vi "Complete_Controller.vi"() -> ()   [LabVIEW 2014]
uses:
  <vilib>/Instr/_visa.llb/VISA Configure Serial Port (Instr).vi
  <vilib>/Utility/file.llb/Read From Spreadsheet File (string).vi
  <vilib>/DAQmx/read.llb/DAQmx Read (Analog 1D DBL NChan 1Samp).vi
  <vilib>/DAQmx/write.llb/DAQmx Write (Analog 1D DBL NChan 1Samp).vi
  <vilib>/DAQmx/write.llb/DAQmx Write (Digital Bool 1Line 1Point).vi
  Environmental Chamber LabVIEW and Instruments/Drivers and Software/keithley_6430/Keithley 6430/Public/Data/Read (Single Point).vi
  Environmental Chamber LabVIEW and Instruments/Drivers and Software/LabVIEW 8.2 Drivers/keithley_24xx/Keithley 24XX/Public/Data/Read (Single Point).vi
  <vilib>/Utility/file.llb/Write To Spreadsheet File (string).vi
  Environmental Chamber LabVIEW and Instruments/Drivers and Software/keithley_24xx/Keithley 24XX/Keithley 24XX.lvlib
  Environmental Chamber LabVIEW and Instruments/Drivers and Software/keithley_6430/Keithley 6430/Keithley 6430.lvlib
panel:
  in  "Turbo pump\nauto on":bool=TRUE
  in  "Use excel file\nfor sequence?":bool
  out "Sequence time left (hrs)":dbl caption="min"
  out "Sequence Preview":cluster{dbl[], dbl[]}[](graph)
  in  "Import sequence file":path
  out "Pressure Control 3":bool caption="Pressure Control"
  in  "valve % open":dbl=100.0 min=0.0 max=100.0 step=5.0
  out "Pressure Control 2":bool caption="Pressure Control"
  out "Keithley 6430":bool
  out "J-Kem":bool caption="J-Kem Temp"
  out "J-Kem Temp (C)":cluster{dbl}(graph)
  out "Keithley 2420":bool caption="Keithley 2430"
  out "Pressure Control":bool
  out "Arduino":bool
  out "temp\n(C)":string
  out "gas\nsensor":string
  out "Arduino humidity (%)":cluster{dbl}(graph)
  out "SRS QCM":bool
  out "MHz":dbl format="%.7f"
  out "Ohm":dbl format="%.4e"
  out "Waveform Chart 7":cluster{dbl, "Resistance out":dbl}(graph)
  out "Chamber Pressure (Torr)":cluster{"f":dbl}(graph)
  in  "Start recording after":dbl caption="min"
  in  "Auto stop after":bool
  in  "hrs":dbl=1000.0 min=0.0
  out "Start Time":string
  out "Elapsed (min)":dbl caption="Elapsed Time (s)"
  in  "Delay between data points (s)":dbl caption="sec" min=0.0 max=30.0 format="%#_13g"
  in  "Vapor\nflow\n(sccm)":sgl(slide) min=0 max=100 step=1 scale=0.0..100.0
  out "Actual":dbl
  out "Boolean 3":bool
  out "Actual":dbl
  out "Boolean":bool
  in  "Gas\nflow\n(sccm)":sgl(slide) min=0 max=100 step=1 scale=0.0..100.0
  in  "Turbo pump auto on":bool
  in  "Desired pressure":dbl min=0.0 max=760.0 step=5.0
  out "Valve position (%)":dbl
  in  "Pressure Control":enum32{"Open Mode (%)", "Pressure Mode (Torr)"}(radio)
  in  "stop":bool
  in  "Experiment Notes":string
  in  "Clear all charts":bool
  out "Save data file path":path
  out "Waveform Chart 2":cluster{"f":dbl, "f":dbl}(graph)
  out "Keithley 2420 (Ohm)":cluster{"Resistance":sgl}(graph)
  out "Keithley 6430 (Ohm)":cluster{"Measurement":dbl}(graph)
  in  "Tab Control":enum32{"Run Sequence", "Create Sequence"}(tab)
  out "User-defined\nsequence 2":string[][](table) caption="Sequence to run"
  in  "Run Sequence":bool
  out "Current step":i32
  out "Step time remaining (min)":dbl caption="min"
  in  "User-defined\nsequence":string[][](table) caption="Create sequence"
  out "QCM mass deposited (ug)":cluster{dbl}(graph)
  in  "rapidox O2 Sensor":bool
  in  "setnag O2 Pump":bool
  in  "Baud Rate 2":i32(ring)=2 items=["2400", "4800", "9600", "19200", "38400", "57600", "115200"]
  in  "Com Port":i32(ring) items=["Com 1", "Com 2", "Com 3", "Com 4", "Com 5", "Com 6", "COM 7", "COM 8", "COM 9", "COM 10", "COM 11", "COM 12", "com 13", "COM 14"]
  in  "Com Port 2":i32(ring) items=["Com 1", "Com 2", "Com 3", "Com 4", "Com 5", "Com 6", "COM 7", "COM 8", "COM 9", "COM 10", "COM 11", "COM 12", "com 13", "COM 14"]
  out "Torr":dbl
  out "%":dbl
  out "atm":dbl
  out "Waveform Chart":cluster{dbl}(graph)
  out "O2 Concentration (PPM)":dbl
  out "Waveform Chart 6":cluster{dbl}(graph)
  # "Currently Unused"
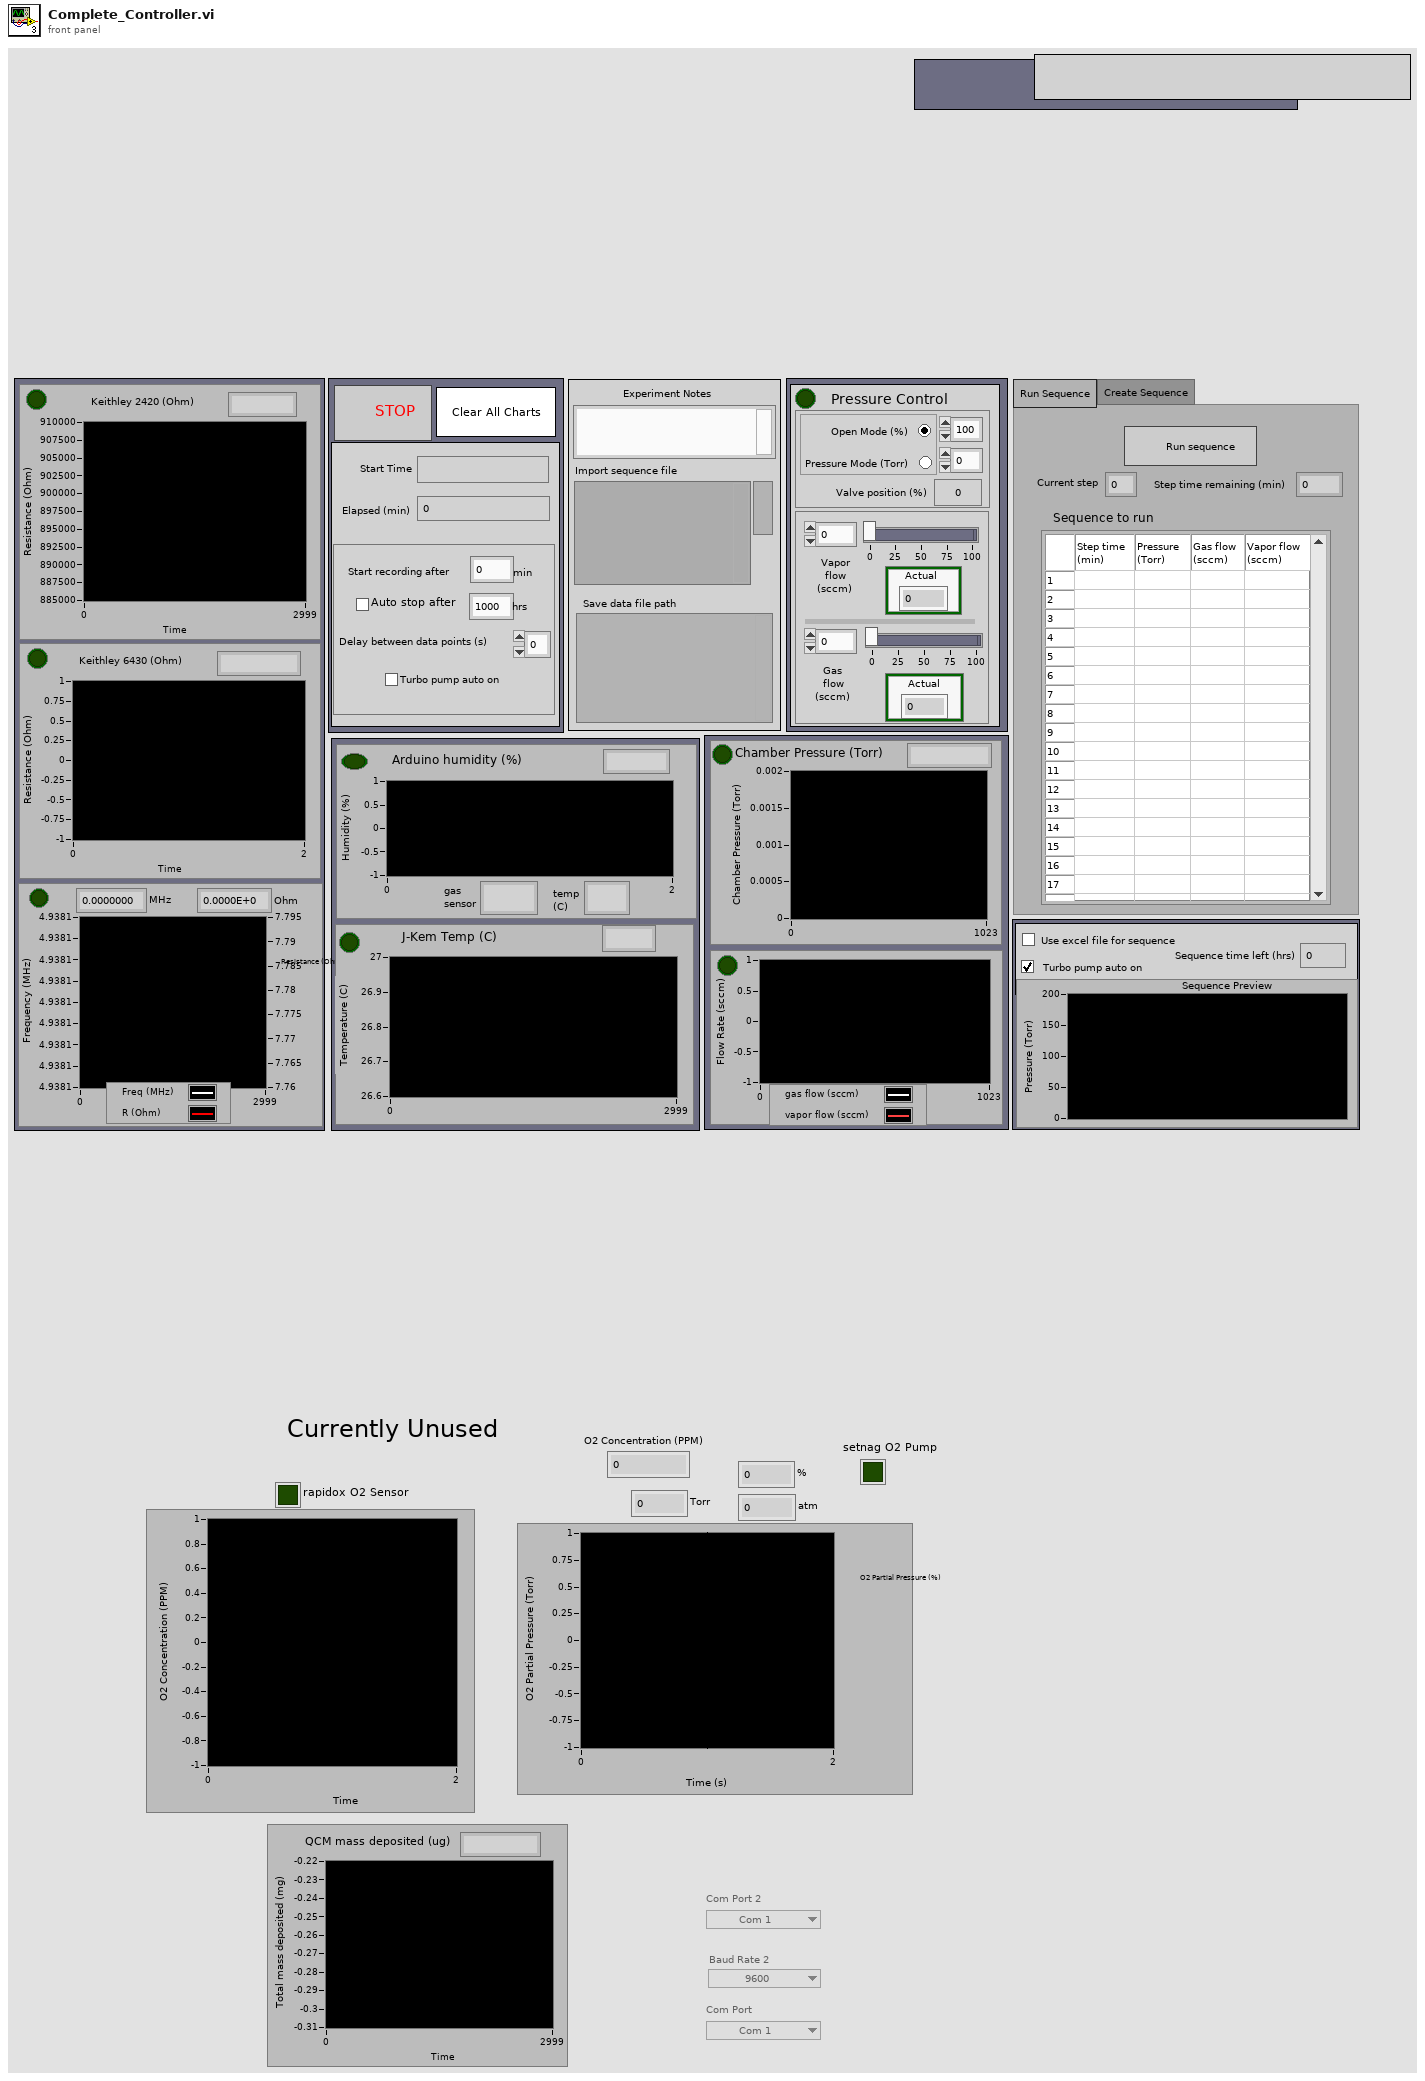
[diagram p1: front panel]
types:
  T1 = enum16{"open", "open or create", "create or replace", "create", "open (read only)"}
  T2 = enum16{"no parity", "odd parity", "even parity", "mark parity", "space parity"}
  T3 = cluster{bool, "VISA resource name":refnum<visa-resource-name>, "error out":errorcluster}
  T4 = cluster{bool, "VISA resource name out":refnum<visa-resource-name>, "error out":errorcluster}
  T5 = cluster{"task out":refnum<k21>, "error out":errorcluster, "task out":refnum<k21>, "error out":errorcluster, "task out":refnum<k21>, "error out":errorcluster, "VISA resource name":refnum<visa-resource-name>, "error out":errorcluster}
  T6 = cluster{"task out":refnum<k21>, "error out":errorcluster, "task out":refnum<k21>, "error out":errorcluster, "task out":refnum<k21>, "error out":errorcluster, "VISA resource name out":refnum<visa-resource-name>, "error out":errorcluster}
  T7 = cluster{bool, "VISA out":refnum<visa-resource-name>, "error out":errorcluster}
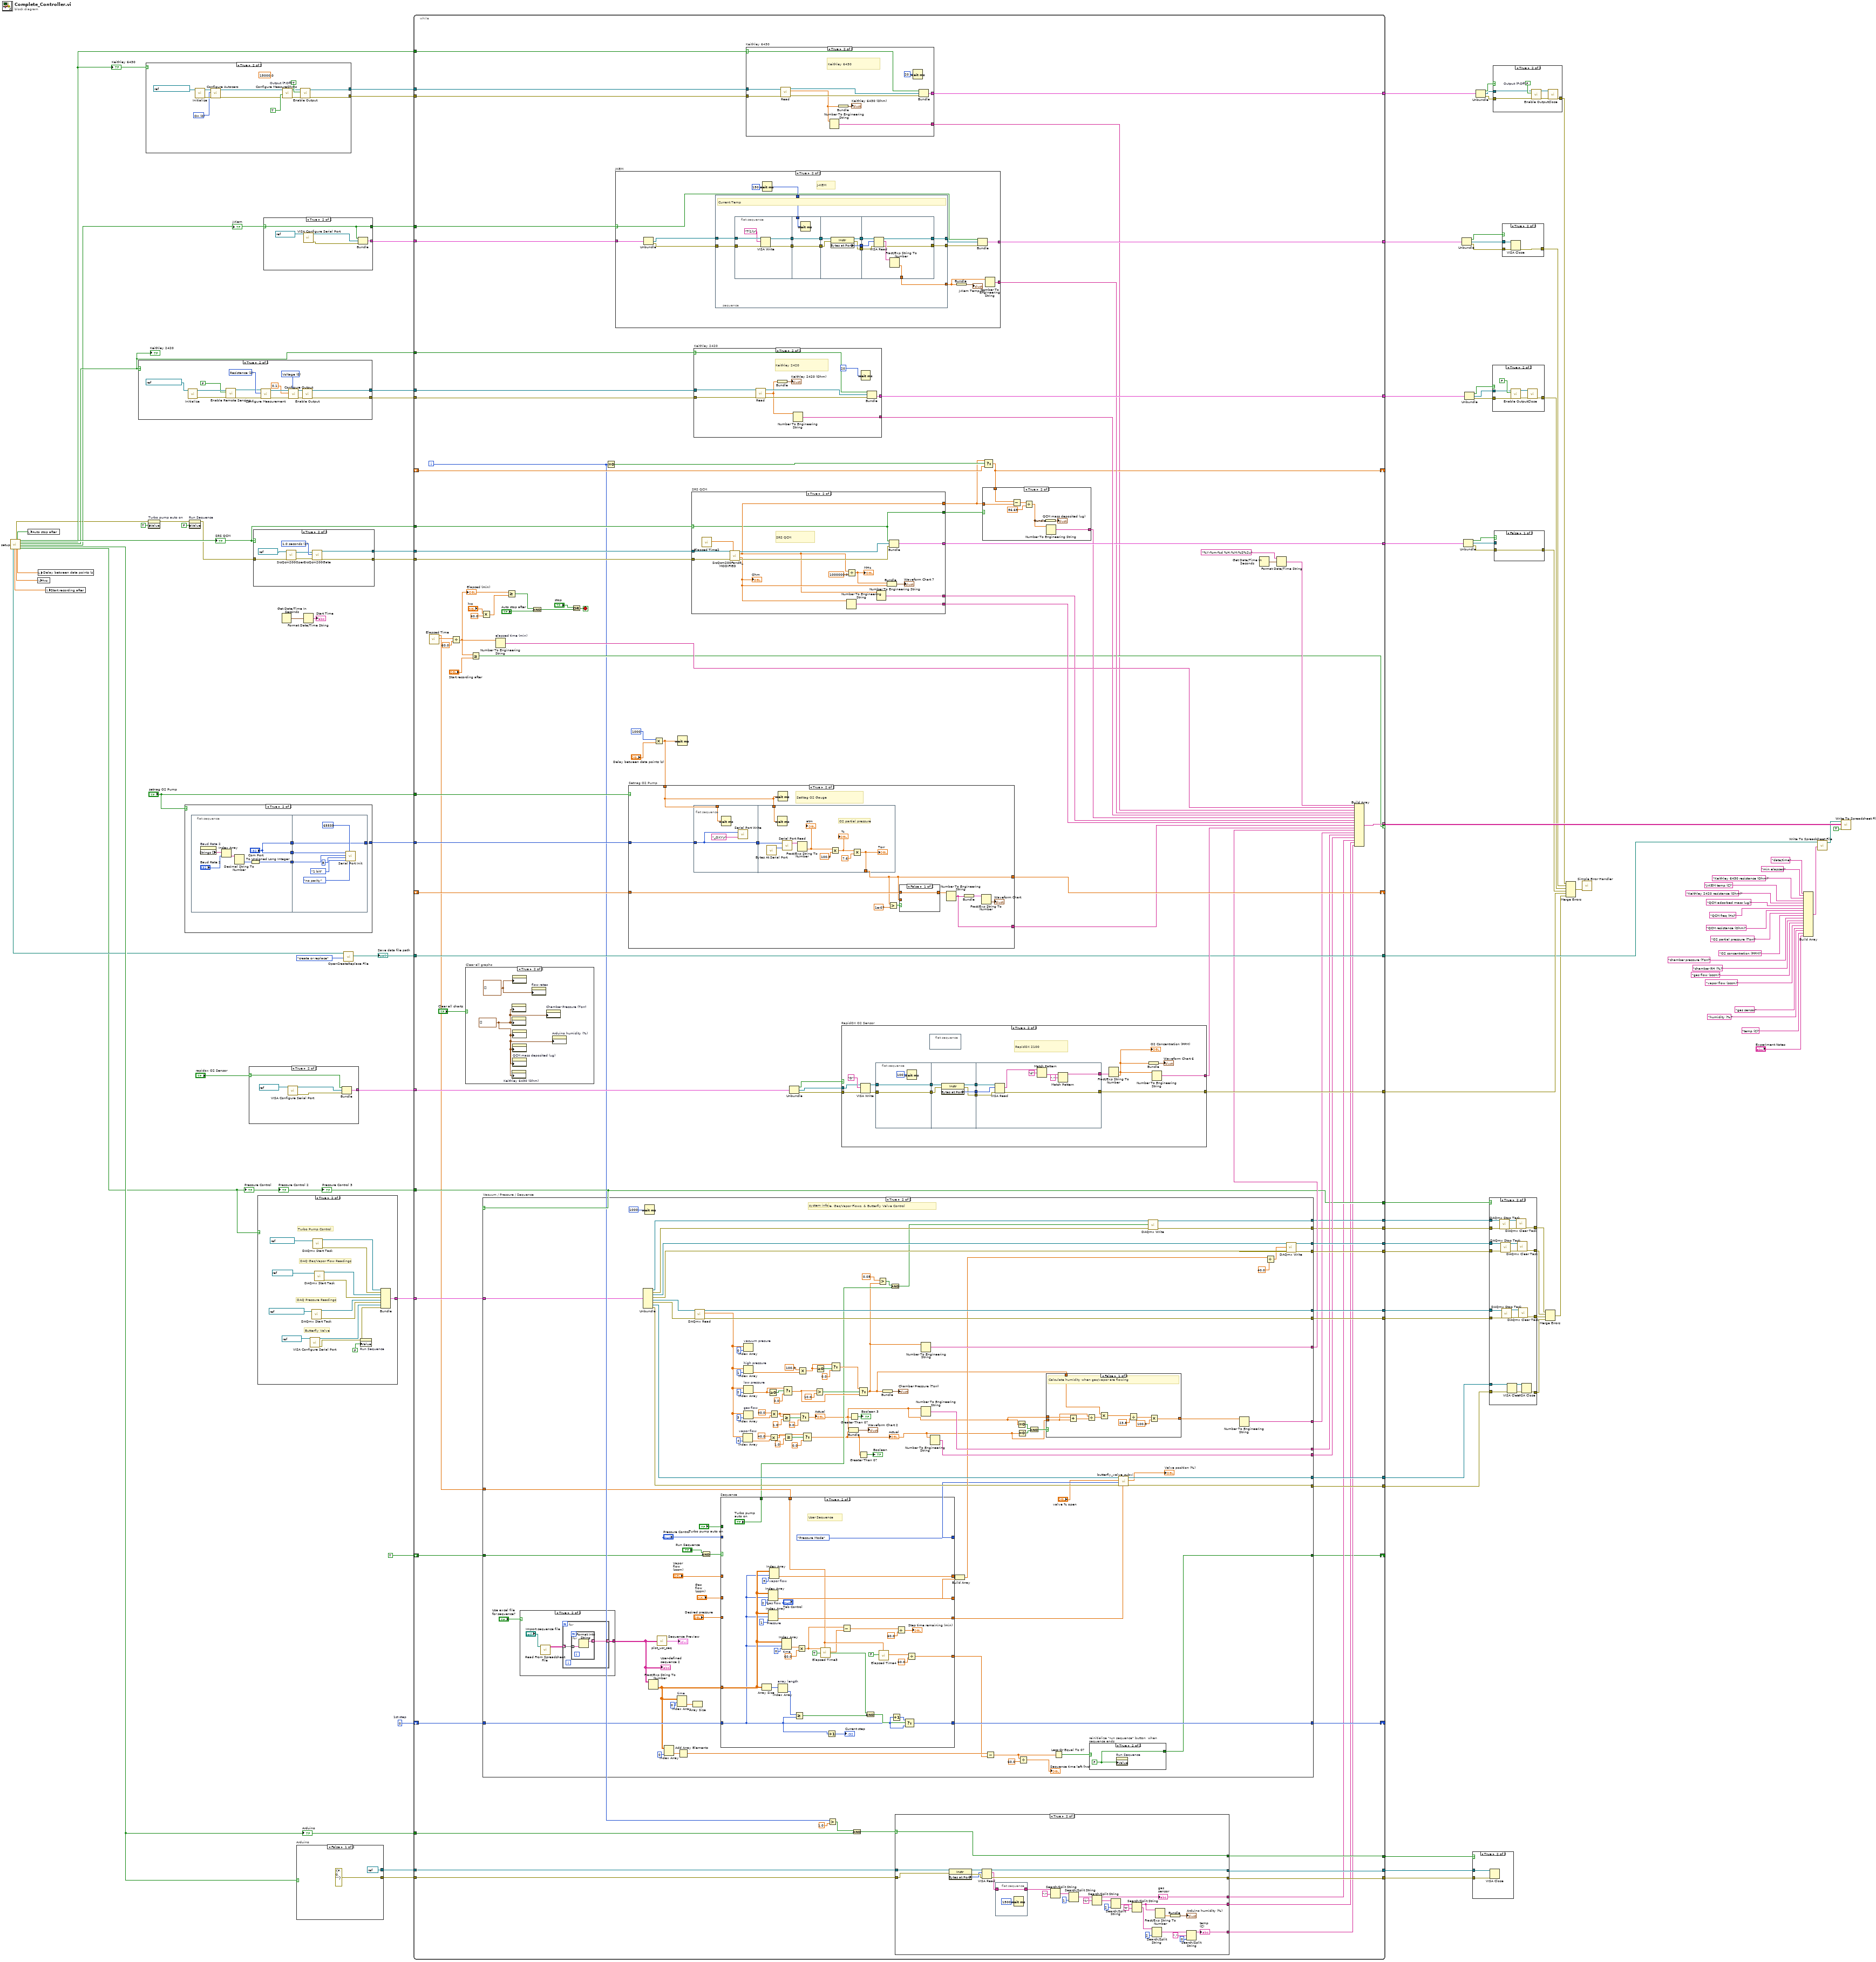
[diagram p0: block diagram]
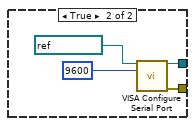
[diagram p3: hidden frame]
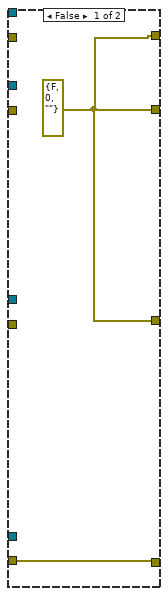
[diagram p4: hidden frame]
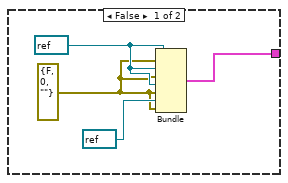
[diagram p5: hidden frame]
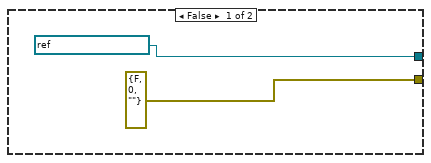
[diagram p7: hidden frame]
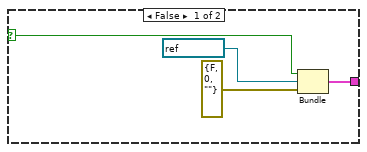
[diagram p8: hidden frame]
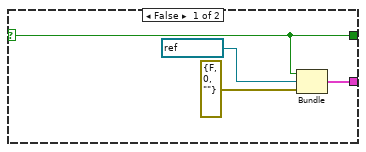
[diagram p10: hidden frame]
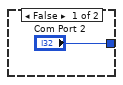
[diagram p11: hidden frame]
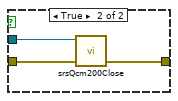
[diagram p12: hidden frame]
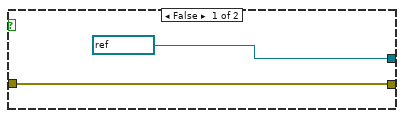
[diagram p13: hidden frame]
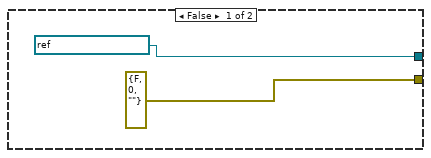
[diagram p15: hidden frame]
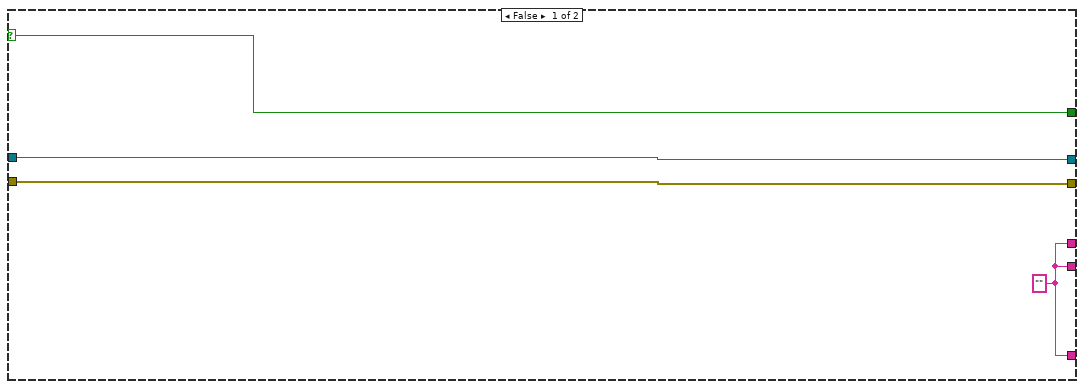
[diagram p16: hidden frame]
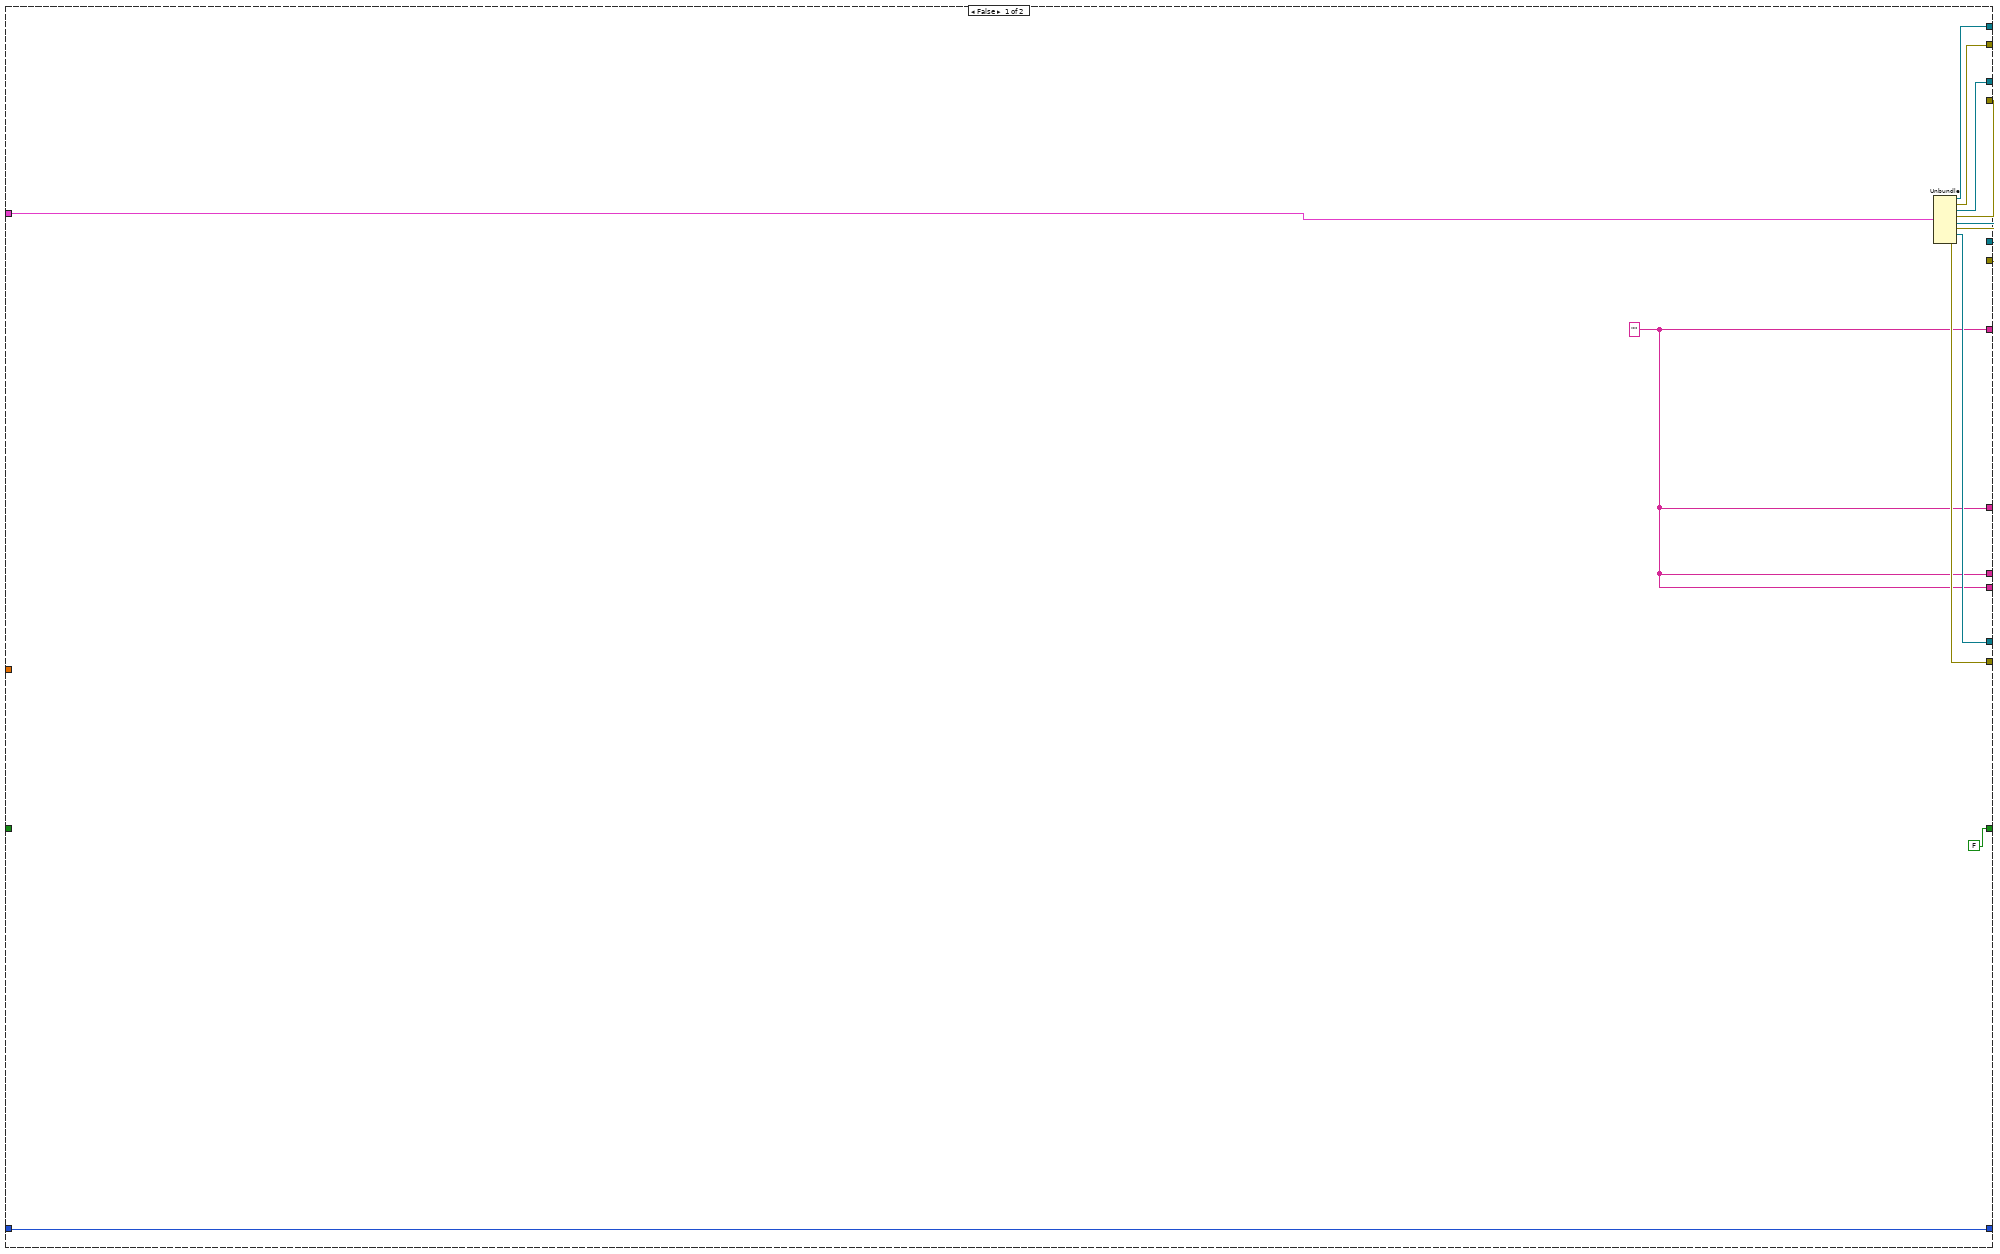
[diagram p17: hidden frame]
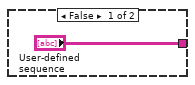
[diagram p18: hidden frame]
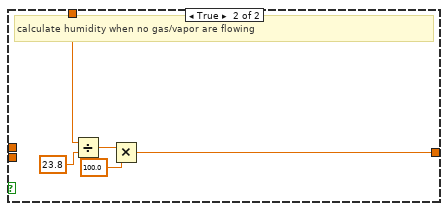
[diagram p19: hidden frame]
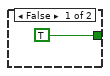
[diagram p20: hidden frame]
diagram:
  w29 = 0  # 1st step
  n1 = call "setup.vi"() -> ("Save file path 2"=w10:path, "begin recording"=w16:dbl, "error IO"=w3:errorcluster, "stop after"=w18:dbl, "Auto Stop 2"=w19:bool, "delay 5"=w17:dbl, "SRS QCM 2"=w15:bool, "Keithley 6431"=w11:bool, "Keithley 2421"=w14:bool, "J-KEM2"=w13:bool, "Arduino2"=w12:bool, "Pressure control 2"=w9:bool)  [unwired: 8 in]
  "SRS QCM" <- w15
  "Arduino" <- w12
  "Pressure Control" <- w9
  "Keithley 2420" <- w14
  "J-Kem" <- w13
  "Keithley 6430" <- w11
  "Pressure Control 2" <- w9
  "Pressure Control 3" <- w9
  n2 = local write "Auto stop after"(w19) -> ()
  n3 = local write "hrs"(w18) -> ()
  n4 = local write "Delay between data points (s)"(w17) -> ()
  n5 = local write "Start recording after"(w16) -> ()
  n6 = case shown="True" w14 {
    tunnel: [refnum<visa-resource-name> "GPIB1::24::INSTR" ("VISA resource name") w108] -> w96
    tunnel: [errorcluster {"status"=FALSE, "code"=0, "source"=""} ("error out") w103] -> w95
    frame False {
    }
    frame True {
      w110 = u16 0 items=["Voltage", "Current"] ("Source Mode  (0: Voltage)")
      w115 = u16 2 items=["Volts", "Current", "Resistance"] ("Function (0: Volts)")
      n7 = call "Initialize.vi"("VISA resource name"=refnum<visa-resource-name> "GPIB1::24::INSTR") -> ("error out"=w104:errorcluster, "VISA resource name out"=w107:refnum<visa-resource-name>)  [unwired: 9 in]
      n8 = call "Enable Remote Sensing.vi"("error in (no error)"=w104, "Enable Remote Sensing (T: Enable)"=FALSE ("4-wire?"), "VISA resource name"=w107) -> ("error out"=w105:errorcluster, "VISA resource name out"=w106:refnum<visa-resource-name>)  [unwired: 7 in]
      n9 = call "Configure Measurement.vi"("error in (no error)"=w105, "Function (0: Volts)"=w115, "VISA resource name"=w106) -> ("error out"=w114:errorcluster, "VISA resource name out"=w113:refnum<visa-resource-name>)  [unwired: 7 in]
      n10 = call "Configure Output.vi"("Source Mode  (0: Voltage)"=w110, "error in (no error)"=w114, "Output Level (0)"=0.1 ("Applied Voltage (V)"), "VISA resource name"=w113) -> ("error out"=w112:errorcluster, "VISA resource name out"=w111:refnum<visa-resource-name>)  [unwired: 6 in]
      n11 = call "Enable Output.vi"("error in (no error)"=w112, "VISA resource name"=w111) -> ("error out"=w103:errorcluster, "VISA resource name out"=w108:refnum<visa-resource-name>)  [unwired: 8 in]
    }
  }
  n12 = case shown="True" w11 {
    tunnel: [refnum<visa-resource-name> "GPIB0::29::INSTR" ("VISA resource name") w125] -> w53
    tunnel: [errorcluster {"status"=FALSE, "code"=0, "source"=""} ("error out") w126] -> w52
    frame False {
    }
    frame True {
      (unwired) 15000.0 ("Resistance Range [Ohms]")
      w121 = u16 0 items=["On", "Off", "Once"] ("Autozero  (0: On)")
      w129 = TRUE  # Output (F:Off)
      n13 = call "Initialize.vi"("VISA resource name"=refnum<visa-resource-name> "GPIB0::29::INSTR") -> ("error out"=w122:errorcluster, "VISA resource name out"=w123:refnum<visa-resource-name>)  [unwired: 4 in, 5 out]
      n14 = call "Configure Autozero.vi"("error in (no error)"=w122, "Autozero  (0: On)"=w121, "VISA resource name"=w123) -> ("error out"=w119:errorcluster, "VISA resource name out"=w120:refnum<visa-resource-name>)  [unwired: 7 in]
      n15 = call "Configure MeasureOhms.vi"("error in (no error)"=w119, "Auto Range (T:Enable)"=TRUE, "VISA resource name"=w120) -> ("error out"=w130:errorcluster, "VISA resource name out"=w128:refnum<visa-resource-name>)  [unwired: 3 in, 4 out]
      n16 = call "Enable Output.vi"("error in (no error)"=w130, "Enable Output (F:Off)"=w129, "VISA resource name"=w128) -> ("error out"=w126:errorcluster, "VISA resource name out"=w125:refnum<visa-resource-name>)  [unwired: 7 out]
    }
  }
  n17 = property on="Turbo pump auto on" class="Bool (strict)"(error in=w3, "Value"=TRUE ("Turbo\npump")) -> (error out=w2:errorcluster)  [unwired: 1 in, 1 out]
  n18 = case shown="True" "setnag O2 Pump" {
    tunnel: ["Com Port 2" w132] -> w92
    frame False {
    }
    frame True {
      n19 = flat-sequence {
        tunnel: ["Com Port"] -> w135
        tunnel: [w137] -> w134
        tunnel: ["Com Port"] -> w133
        tunnel: w135 -> [w143]
        tunnel: w134 -> [w142]
        tunnel: w133 -> [w144]
        tunnel: [w144] -> w132
        frame #0 {
          n20 = property on="Baud Rate 2" class="Ring (strict)"() -> ("Strings []"=w139:string[])  [unwired: 2 in, 2 out]
          n21 = Index Array(array=w139, index="Baud Rate 2") -> (element=w140:string)
          n22 = Decimal String To Number(string=w140) -> (number=w138:i32)  [unwired: 2 in, 1 out]
          n23 = To Unsigned Long Integer(number=w138) -> (unsigned 32bit integer=w137:u32)
        }
        frame #1 {
          n24 = call <vilib>:"Serial Port Init.vi"("parity"=T2."no parity", "buffer size"=u16 65535, "stop bits"=enum16{"1 bit", "1.5 bits", "2 bits"}."1 bit", "data bits"=u16 8, "baud rate"=w142, "port number"=w143) -> ()  [unwired: 1 in, 1 out]
        }
      }
    }
  }
  n25 = property on="Run Sequence" class="Bool (strict)"(error in=w2, "Value"=FALSE ("Run Sequence")) -> (error out=w7:errorcluster)  [unwired: 1 in, 1 out]
  n26 = case shown="True" "rapidox O2 Sensor" {
    selector: "rapidox O2 Sensor" -> [w149 w154]
    tunnel: [w150 w155] -> w63
    frame False {
      n27 = Bundle(w149, "VISA resource name"=refnum<visa-resource-name> "COM7", "error out"=errorcluster {"status"=FALSE, "code"=0, "source"=""}) -> (w150:T3)  [unwired: 1 in]
    }
    frame True {
      n28 = call-poly "VISA Configure Serial Port"("VISA resource name"=refnum<visa-resource-name> "COM7") -> ("VISA resource name out"=w156:refnum<visa-resource-name>, "error out"=w153:errorcluster)  [unwired: 13 in]
      n29 = Bundle(w154, "VISA resource name out"=w156, "error out"=w153) -> (w155:T4)  [unwired: 1 in]
    }
  }
  n30 = case shown="True" w15 {
    tunnel: [refnum<visa-resource-name> "COM6" ("VISA in") w162] -> w94
    tunnel: [w158 w161] -> w93
    tunnel: w7 -> [w158 w160]
    frame False {
    }
    frame True {
      w166 = u16 1 items=["0.1 seconds", "1.0 seconds", "10.0 seconds"] ("Gate in")
      n31 = call "SrsQcm200Open.vi"("error in"=w160, "VISA in"=refnum<visa-resource-name> "COM6") -> ("error out"=w163:errorcluster, "VISA out"=w164:refnum<visa-resource-name>)  [unwired: 3 in]
      n32 = call "SrsQcm200Gate.vi"("VISA in"=w164, "Gate in"=w166, "error in (no error)"=w163) -> ("VISA out"=w162:refnum<visa-resource-name>, "error out"=w161:errorcluster)  [unwired: 14 in, 1 out]
    }
  }
  n33 = case shown="True" w9 {
    tunnel: [w167 w174] -> w34
    frame False {
      w169 = refnum<k21> refnum ("task out")
      w168 = errorcluster {"status"=FALSE, "code"=0, "source"=""} ("error out")
      n34 = Bundle("task out"=w169, "error out"=w168, "task out"=w169, "error out"=w168, "task out"=w169, "error out"=w168, "VISA resource name"=refnum<visa-resource-name> refnum, "error out"=w168) -> (w167:T5)  [unwired: 1 in]
    }
    frame True {
      # "Turbo Pump Control"
      # "DAQ Gas/Vapor Flow Readings"
      # "DAQ Pressure Readings"
      # "Butterfly Valve"
      n35 = call-poly "VISA Configure Serial Port"("VISA resource name"=refnum<visa-resource-name> "COM5") -> ("VISA resource name out"=w175:refnum<visa-resource-name>, "error out"=w171:errorcluster)  [unwired: 13 in]
      n36 = call <vilib>:"DAQmx Start Task.vi"("task/channels in"=refnum<k21> "AllDaqReadings") -> ("task out"=w177:refnum<k21>, "error out"=w176:errorcluster)  [unwired: 13 in]
      n37 = call <vilib>:"DAQmx Start Task.vi"("task/channels in"=refnum<k21> "TurboON") -> ("task out"=w181:refnum<k21>, "error out"=w180:errorcluster)  [unwired: 13 in]
      n38 = call <vilib>:"DAQmx Start Task.vi"("task/channels in"=refnum<k21> "Setflow") -> ("task out"=w179:refnum<k21>, "error out"=w178:errorcluster)  [unwired: 13 in]
      n39 = property on="Run Sequence" class="Bool (strict)"(error in=w171, "Value"=FALSE ("Run Sequence")) -> (error out=w173:errorcluster)  [unwired: 1 in, 1 out]
      n40 = Bundle("task out"=w181, "error out"=w180, "task out"=w179, "error out"=w178, "task out"=w177, "error out"=w176, "VISA resource name out"=w175, "error out"=w173) -> (w174:T6)  [unwired: 1 in]
    }
  }
  n41 = case shown="True" w13 {
    selector: w13 -> [w186 w191]
    tunnel: [w187 w192] -> w81
    tunnel: [w186 w191] -> w75
    frame False {
      n42 = Bundle(w186, "VISA resource name"=refnum<visa-resource-name> "COM3", "error out"=errorcluster {"status"=FALSE, "code"=0, "source"=""}) -> (w187:T3)  [unwired: 1 in]
    }
    frame True {
      n43 = call-poly "VISA Configure Serial Port"("VISA resource name"=refnum<visa-resource-name> "COM3") -> ("VISA resource name out"=w193:refnum<visa-resource-name>, "error out"=w190:errorcluster)  [unwired: 13 in]
      n44 = Bundle(w191, "VISA resource name out"=w193, "error out"=w190) -> (w192:T4)  [unwired: 1 in]
    }
  }
  n45 = Get Date/Time In Seconds() -> (seconds since 1Jan1904=w99:timestamp)
  n46 = case "Arduino" shown="False" w12 {
    tunnel: [refnum<visa-resource-name> refnum ("VISA resource name out") w200] -> w28
    tunnel: [errorcluster {"status"=FALSE, "code"=0, "source"=""} ("error out") w197] -> w27
    frame False {
    }
    frame True {
      n47 = call-poly "VISA Configure Serial Port"("VISA resource name"=refnum<visa-resource-name> "COM12", "baud rate (9600)"=u32 9600) -> ("VISA resource name out"=w200:refnum<visa-resource-name>, "error out"=w197:errorcluster)  [unwired: 12 in]
    }
  }
  n48 = Format Date/Time String(seconds (now)=w99) -> (date/time string=→"Start Time":string)  [unwired: 2 in]
  n49 = call "OpenCreateReplace File.vi"("function (open:0)"=T1."create or replace", "file path"=w10) -> ("new file path"=w20:path)  [unwired: 6 in, 3 out]
  "Save data file path" <- w20
  n50 = while {
    shift-right: [w290] -> _
    shift-left: _ -> [w289]
    tunnel: [w219] -> w97 mode=indexing if=w218
    tunnel: w14 -> [w258]
    tunnel: w96 -> [w287]
    tunnel: w95 -> [w286]
    tunnel: w94 -> [w285]
    tunnel: w93 -> [w284]
    tunnel: w15 -> [w282]
    tunnel: "setnag O2 Pump" -> [w275]
    tunnel: w92 -> [w281]
    tunnel: [w277] -> w89
    tunnel: [w276] -> w85
    tunnel: w81 -> [w274]
    tunnel: [w273] -> w80
    tunnel: w75 -> [w271]
    tunnel: w63 -> [w267]
    tunnel: [w262] -> w61
    tunnel: [w257] -> w60
    tunnel: w20 -> [w257]
    shift-right: [w240] -> _
    shift-left: _ -> [w242]
    tunnel: w53 -> [w254]
    tunnel: w52 -> [w253]
    tunnel: [w252] -> w51
    tunnel: w11 -> [w251]
    tunnel: w9 -> [w232]
    tunnel: [w248] -> w47
    tunnel: [w247] -> w44
    tunnel: [w246] -> w46
    tunnel: [w245] -> w45
    tunnel: [w232] -> w43
    tunnel: [w244] -> w38
    tunnel: w34 -> [w236]
    tunnel: [w235] -> w32
    tunnel: [w234] -> w31
    tunnel: [w233] -> w30
    shift-right: [w231] -> _
    shift-left: w29 -> [w230]
    tunnel: w12 -> [w215]
    tunnel: w28 -> [w225]
    tunnel: w27 -> [w224]
    tunnel: [w223] -> w26
    tunnel: [w222] -> w25
    tunnel: [w221] -> w24
    shift-right: [w206] -> _
    shift-left: TRUE -> [w207]
    i -> [w204]
    stop <- w270 stop-if-true
    n51 = call "Elapsed Time"() -> ("Present (s)"=w229:dbl, "Elapsed Time (s)"=w269:dbl)  [unwired: 12 in, 6 out]
    n52 = Divide(x=w269, y=60.0) -> (x/y=w209:dbl)
    "Elapsed (min)" <- w209
    n53 = case "Clear all graphs" shown="True" "Clear all charts" {
      frame False {
      }
      frame True {
        w529 = cluster{dbl, "Resistance out":dbl}[] [] ("History Data")
        w528 = cluster{dbl}[] [] ("History Data")
        n54 = property on="Keithley 2420 (Ohm)" class="WFChart (strict)"("History Data"=w528) -> ()  [unwired: 2 in, 2 out]
        n55 = property on="J-Kem Temp (C)" class="WFChart (strict)"("History Data"=w528) -> ()  [unwired: 2 in, 2 out]
        n56 = property on="Keithley 6430 (Ohm)" class="WFChart (strict)"("History Data"=w528) -> ()  [unwired: 2 in, 2 out]
        n57 = property on="Waveform Chart 7" class="WFChart (strict)"("History Data"=w529) -> ()  [unwired: 2 in, 2 out]
        n58 = property on="Waveform Chart" class="WFChart (strict)"("History Data"=w528) -> ()  [unwired: 2 in, 2 out]
        n59 = property on="Waveform Chart 6" class="WFChart (strict)"("History Data"=w528) -> ()  [unwired: 2 in, 2 out]
        n60 = property on="QCM mass deposited (ug)" class="WFChart (strict)"("History Data"=w528) -> ()  [unwired: 2 in, 2 out]
        n61 = property on="flow rates" class="WFChart (strict)"("History Data"=w529) -> ()  [unwired: 2 in, 2 out]
        n62 = property on="Chamber Pressure (Torr)" class="WFChart (strict)"("History Data"=w528) -> ()  [unwired: 2 in, 2 out]
        n63 = property on="Arduino humidity (%)" class="WFChart (strict)"("History Data"=w528) -> ()  [unwired: 2 in, 2 out]
      }
    }
    n64 = Greater Or Equal?(x=w209, y="Start recording after") -> (x >= y?=w218:bool)
    n65 = Multiply(x="hrs", y=60.0) -> (x*y=w201:dbl)
    n66 = case "Vacuum / Pressure / Sequence" shown="True" w232 {
      tunnel: [w332 w439] -> w247
      tunnel: [w333 w438] -> w245
      tunnel: [w335 w419] -> w248
      tunnel: [w334 w420] -> w246
      tunnel: [w333 w410] -> w244
      tunnel: [w328 w400] -> w239
      tunnel: [w328 w399] -> w238
      tunnel: [w328 w397] -> w237
      tunnel: w236 -> [w338 w395]
      tunnel: [w337 w386] -> w235
      tunnel: [w336 w385] -> w234
      tunnel: [w331 w384] -> w233
      tunnel: w230 -> [w330 w366]
      tunnel: [w330 w381] -> w231
      tunnel: w229 -> [_ w380]
      tunnel: w207 -> [_ w357]
      tunnel: [FALSE ("new element/subarray") w352] -> w206
      tunnel: [w328 w351] -> w205
      frame False {
        w328 = ""
        n67 = Unbundle(w338) -> ("task out"=w337:refnum<k21>, "error out"=w336:errorcluster, "task out"=w335:refnum<k21>, "error out"=w334:errorcluster, "task out"=w332:refnum<k21>, "error out"=w333:errorcluster, "VISA resource name out"=w331:refnum<visa-resource-name>)  [unwired: 1 out]
      }
      frame True {
        # "system info"
        # "DAQ Pressure, Gas/Vapor Flows, & Butterfly Valve Control"
        n68 = case shown="True" "Use excel file\nfor sequence?" {
          tunnel: ["User-defined\nsequence" w442] -> w343
          frame False {
          }
          frame True {
            n69 = call-poly <vilib>:"Read From Spreadsheet File.vi"("file path (dialog if empty)"="Import sequence file") -> ("all rows"=w444:string[][])  [unwired: 6 in, 4 out]
            n70 = for {
              tunnel: w444 -> [w446] mode=indexing
              tunnel: [w445] -> w442 mode=indexing
              n71 = for {
                tunnel: w446 -> [w448] mode=indexing
                tunnel: [w447] -> w445 mode=indexing
                n72 = Format Into String(w448) -> (resulting string=w447:string)  [unwired: 3 in, 1 out]
              }
            }
          }
        }
        "User-defined\nsequence 2" <- w343
        n73 = Unbundle(w395) -> ("task out"=w388:refnum<k21>, "error out"=w387:errorcluster, "task out"=w389:refnum<k21>, "error out"=w390:errorcluster, "task out"=w391:refnum<k21>, "error out"=w392:errorcluster, "VISA resource name out"=w393:refnum<visa-resource-name>, "error out"=w394:errorcluster)
        n74 = Wait (ms)(milliseconds to wait=u32 1000) -> ()  [unwired: 1 out]
        n75 = Fract/Exp String To Number(string=w343) -> (number=w356:dbl[][])  [unwired: 3 in, 1 out]
        n76 = call "plot_usr_seq.vi"("User-defined sequence"=w343) -> ("Sequence Preview"=→"Sequence Preview":cluster{dbl[], dbl[]}[])
        n77 = Index Array(array=w356, index (col)=0 ("disabled index (col)")) -> (element=w370:dbl[])  [unwired: 1 in]
        n78 = Index Array "time"(array=w356, index (row)=0 ("disabled index (col)")) -> (element=w355:dbl[])  [unwired: 1 in]
        n79 = Add Array Elements(numeric array=w370) -> (sum=w361:dbl)
        n80 = Array Size(array=w355) -> ()  [unwired: 1 out]
        n81 = call-poly <vilib>:"DAQmx Read.vi"("task/channels in"=w391, "error in"=w392) -> ("task out"=w439:refnum<k21>, "data"=w430:dbl[], "error out"=w438:errorcluster)  [unwired: 11 in]
        n82 = And(x="Run Sequence", y=w357) -> (x .and. y?=w358:bool)
        n83 = case "Sequence" shown="True" w358 {
          tunnel: w380 -> [_ w487]
          tunnel: [w472 w488] -> w381
          tunnel: w366 -> [w472 w474]
          tunnel: "Vapor\nflow\n(sccm)" -> [w471 _]
          tunnel: "Gas\nflow\n(sccm)" -> [w470 _]
          tunnel: [w471 w496] -> w377
          tunnel: [w470 w495] -> w376
          tunnel: [w468 w494] -> w362
          tunnel: "Desired pressure" -> [w468 _]
          tunnel: "Turbo pump auto on" -> [w469 _]
          tunnel: [w469 "Turbo pump\nauto on"] -> w372
          tunnel: w356 -> [_ w481]
          tunnel: "Pressure Control" -> [w467 _]
          tunnel: [w467 enum32{"Open Mode", "Pressure Mode"}."Pressure Mode" ("Pressure Control")] -> w367
          tunnel: [0.0 w484] -> w360
          frame False {
          }
          frame True {
            # "User Sequence"
            n84 = Array Size(array=w481) -> (size(s)=w504:i32[])
            n85 = Index Array "gas flow"(array=w481, index (row)=w474, index (col)=2 ("disabled index (col)")) -> (element=w495:dbl)
            n86 = Index Array "Pressure"(array=w481, index (row)=w474, index (col)=1 ("disabled index (col)")) -> (element=w494:dbl)
            n87 = Index Array "vapor flow"(array=w481, index (row)=w474, index (col)=3 ("disabled index (col)")) -> (element=w496:dbl)
            n88 = Index Array "array length"(array=w504) -> (element=w482:i32)  [unwired: 1 in]
            n89 = Index Array "time"(array=w481, index (row)=w474, index (col)=0) -> (element=w493:dbl)
            n90 = Greater Or Equal?(x=w482, y=w474) -> (x >= y?=w501:bool)
            n91 = Multiply(x=w493, y=60.0) -> (x*y=w479:dbl)
            n92 = call "Elapsed Time3"("Time Target (s)"=w479, "Auto Reset"=TRUE, "Set Start Time (s)"=w487) -> ("Elapsed Time (s)"=w478:dbl, "Time has Elapsed"=w500:bool)  [unwired: 9 in, 6 out]
            n93 = Increment(x=w474) -> (x+1=→"Current step":i32)
            n94 = Subtract(x=w479, y=w478) -> (x-y=w475:dbl)
            n95 = And(x=w500, y=w501) -> (x .and. y?=w490:bool)
            n96 = call "Elapsed Time4"("Reset"=FALSE, "Set Start Time (s)"=w487) -> ("Elapsed Time (s)"=w485:dbl)  [unwired: 10 in, 7 out]
            n97 = Increment(x=w474) -> (x+1=w489:i32)
            n98 = Divide(x=w475, y=60.0) -> (x/y=→"Step time remaining (min)":dbl)
            n99 = Select(t=w489, s=w490, f=w474) -> (s? t:f=w488:i32)
            n100 = Divide(x=w485, y=60.0) -> (x/y=w484:dbl)
          }
        }
        n101 = Index Array "vapor flow"(array=w430, index=4) -> (element=w426:dbl)
        n102 = Index Array "vacuum presure"(array=w430, index=0) -> ()  [unwired: 1 out]
        n103 = Index Array "high pressure"(array=w430, index=1) -> (element=w433:dbl)
        n104 = Index Array "low pressure"(array=w430, index=2) -> (element=w404:dbl)
        n105 = Index Array "gas flow"(array=w430, index=3) -> (element=w428:dbl)
        n106 = Greater Or Equal To 0?(x=w404) -> (x >= 0?=w405:bool)
        n107 = Multiply(x=40.0, y=w426) -> (x*y=w417:dbl)
        n108 = Multiply(x=40.0, y=w428) -> (x*y=w414:dbl)
        n109 = Greater Or Equal?(x=w414, y=1.0) -> (x >= y?=w413:bool)
        n110 = Select(t=w404, s=w405, f=0.0) -> (s? t:f=w403:dbl)
        n111 = Greater Or Equal?(x=w417, y=1.0) -> (x >= y?=w416:bool)
        n112 = Multiply(x=100.0, y=w433) -> (x*y=w421:dbl)
        n113 = Select(t=w414, s=w413, f=0.0) -> (s? t:f=w345:dbl)
        "Actual" <- w345
        n114 = Select(t=w417, s=w416, f=0.0) -> (s? t:f=w344:dbl)
        "Actual" <- w344
        n115 = Greater?(x=w403, y=10.0) -> (0:w409:bool)
        n116 = Greater Or Equal To 0?(x=w421) -> (x >= 0?=w423:bool)
        n117 = Select(t=w421, s=w423, f=0.0) -> (s? t:f=w408:dbl)
        n118 = Bundle("f"=w345, "f"=w344) -> (→"Waveform Chart 2":cluster{"f":dbl, "f":dbl})  [unwired: 1 in]
        n119 = Greater Than 0?(x=w345) -> (x > 0?=→"Boolean 3":bool)
        n120 = Select(t=w408, s=w409, f=w403) -> (s? t:f=w347:dbl)
        n121 = Greater Than 0?(x=w344) -> (x > 0?=→"Boolean":bool)
        n122 = Greater?(x=0.05, y=w347) -> (0:w371:bool)
        n123 = Bundle("f"=w347) -> (→"Chamber Pressure (Torr)":cluster{"f":dbl})  [unwired: 1 in]
        n124 = And(x=w371, y=w372) -> (x .and. y?=w382:bool)
        n125 = Number To Engineering String(4:w345) -> (0:w399:string)  [unwired: 3 in]
        n126 = Number To Engineering String(4:w347) -> (0:w400:string)  [unwired: 3 in]
        n127 = Number To Engineering String(4:w344) -> (0:w397:string)  [unwired: 3 in]
        n128 = Build Array(w377, w376) -> (w375:dbl[])
        n129 = Subtract(x=w361, y=w360) -> (x-y=w340:dbl)
        n130 = Equal To 0?(x=w345) -> (x = 0?=w349:bool)
        n131 = Equal To 0?(x=w344) -> (x = 0?=w350:bool)
        n132 = Divide(x=w340, y=60.0) -> (x/y=→"Sequence time left (hrs)":dbl)
        n133 = And(x=w349, y=w350) -> (x .and. y?=w348:bool)
        n134 = case shown="False" w348 {
          tunnel: w347 -> [w450 w460]
          tunnel: [w449 w459] -> w346
          tunnel: w345 -> [w458 _]
          tunnel: w344 -> [w456 _]
          frame False {
            # "Calculate humidity when gas/vapor are flowing"
            n135 = Add(x=w458, y=w456) -> (x+y=w457:dbl)
            n136 = Divide(x=w456, y=w457) -> (x/y=w451:dbl)
            n137 = Multiply(x=w450, y=w451) -> (x*y=w452:dbl)
            n138 = Divide(x=w452, y=23.8) -> (x/y=w454:dbl)
            n139 = Multiply(x=w454, y=100.0) -> (x*y=w449:dbl)
          }
          frame True {
            # "calculate humidity when no gas/vapor are flowing"
            n140 = Divide(x=w460, y=23.8) -> (x/y=w462:dbl)
            n141 = Multiply(x=w462, y=100.0) -> (x*y=w459:dbl)
          }
        }
        n142 = Less Or Equal To 0?(x=w340) -> (x <= 0?=w353:bool)
        n143 = case "reinitialize \"run sequence\" button  when sequence ends" shown="True" w353 {
          tunnel: [TRUE ("Run Sequence") w465] -> w352
          frame False {
          }
          frame True {
            w465 = FALSE ("Run Sequence")
            n144 = property on="Run Sequence" class="Bool (strict)"("Value"=w465) -> ()  [unwired: 2 in, 2 out]
          }
        }
        n145 = call "butterfly_valve_subvi.vi"("Desired pressure"=w362, "error in (no error)"=w394, "Pressure Control"=w367, 10:"valve % open", "VISA Refnum in"=w393) -> ("error out"=w410:errorcluster, "Valve position (%)"=→"Valve position (%)":dbl, "VISA Refnum out"=w384:refnum<visa-resource-name>)  [unwired: 4 in]
        n146 = call-poly <vilib>:"DAQmx Write.vi"("task/channels in"=w388, "data"=w382, "error in"=w387) -> ("task out"=w386:refnum<k21>, "error out"=w385:errorcluster)  [unwired: 10 in, 1 out]
        n147 = Number To Engineering String(4:w346) -> (0:w351:string)  [unwired: 3 in]
        n148 = Divide(x=w375, y=40.0 ("Waveform")) -> (x/y=w412:dbl[])
        n149 = call-poly <vilib>:"DAQmx Write.vi"("task/channels in"=w389, "data"=w412, "error in"=w390) -> ("task out"=w419:refnum<k21>, "error out"=w420:errorcluster)  [unwired: 10 in, 1 out]
      }
    }
    n150 = Number To Engineering String "elapsed time (min)"(4:w209) -> (0:w291:string)  [unwired: 3 in]
    n151 = Greater Or Equal?(x=w209, y=w201) -> (x >= y?=w212:bool)
    n152 = And(x=w212, y="Auto stop after") -> (x .and. y?=w210:bool)
    n153 = Or(x="stop", y=w210) -> (x .or. y?=w270:bool)
    n154 = Equal To 0?(x=w204) -> (x = 0?=w243:bool)
    n155 = case "JKEM" shown="True" w271 {
      selector: w271 -> [_ w567]
      tunnel: w274 -> [w565 w572]
      tunnel: [w565 w570] -> w273
      tunnel: ["" w568] -> w272
      frame False {
      }
      frame True {
        w576 = u32 150 ("milliseconds to wait")
        # "J-KEM"
        n156 = Unbundle(w572) -> ("VISA resource name out"=w571:refnum<visa-resource-name>, "error out"=w566:errorcluster)  [unwired: 1 out]
        n157 = stacked-sequence {
          tunnel: w571 -> [w582]
          tunnel: w566 -> [w581]
          tunnel: w576 -> [w580]
          tunnel: [w578] -> w573
          tunnel: [w577] -> w574
          tunnel: [w579] -> w569
          frame #0 {
            # "Current Temp"
            n158 = flat-sequence {
              tunnel: w582 -> [w594]
              tunnel: w581 -> [w593]
              tunnel: [w591] -> w589
              tunnel: [w590] -> w588
              tunnel: w580 -> [w597]
              tunnel: [w596] -> w587
              tunnel: w589 -> [w596]
              tunnel: w588 -> [w595]
              tunnel: [w595] -> w586
              tunnel: w587 -> [w602]
              tunnel: w586 -> [w601]
              tunnel: [w600] -> w585
              tunnel: [w599] -> w584
              tunnel: [w598] -> w583
              tunnel: w585 -> [w609]
              tunnel: w584 -> [w608]
              tunnel: w583 -> [w607]
              tunnel: [w604] -> w577
              tunnel: [w605] -> w578
              tunnel: [w603] -> w579
              frame #0 {
                n159 = VISA Write(VISA resource name=w594, write buffer="T(1)\r", error in (no error)=w593) -> (VISA resource name out=w591:refnum<visa-resource-name>, error out=w590:errorcluster)  [unwired: 1 out]
              }
              frame #1 {
                n160 = Wait (ms)(milliseconds to wait=w597) -> ()  [unwired: 1 out]
              }
              frame #2 {
                n161 = property class="Instr"(reference=w602, error in=w601) -> (reference out=w600:refnum<visa-resource-name>, error out=w598:errorcluster, "Bytes at Port"=w599:u32)
              }
              frame #3 {
                n162 = VISA Read(VISA resource name=w609, byte count=w608, error in (no error)=w607) -> (VISA resource name out=w605:refnum<visa-resource-name>, read buffer=w606:string, error out=w604:errorcluster)  [unwired: 1 out]
                n163 = Fract/Exp String To Number(string=w606) -> (number=w603:dbl)  [unwired: 3 in, 1 out]
              }
            }
          }
        }
        n164 = Wait (ms)(milliseconds to wait=w576) -> ()  [unwired: 1 out]
        n165 = Bundle(w569) -> (→"J-Kem Temp (C)":cluster{dbl})  [unwired: 1 in]
        n166 = Bundle(w567, "VISA resource name out"=w573, "error out"=w574) -> (w570:T4)  [unwired: 1 in]
        n167 = Number To Engineering String(4:w569) -> (0:w568:string)  [unwired: 3 in]
      }
    }
    n168 = Multiply(x=u32 1000, y="Delay between data points (s)") -> (x*y=w261:dbl)
    n169 = case "Setnag O2 Pump" shown="True" w275 {
      tunnel: [w646 w650] -> w290
      tunnel: w289 -> [w646 w651]
      tunnel: w261 -> [_ w647]
      tunnel: w281 -> [_ w649]
      tunnel: ["" w648] -> w280
      frame False {
      }
      frame True {
        # "SetNag O2 Gauge"
        n170 = flat-sequence {
          tunnel: [w660] -> w657
          tunnel: w647 -> [w662]
          tunnel: w649 -> [w660]
          tunnel: w657 -> [w663]
          tunnel: w647 -> [w670]
          tunnel: [w666] -> w650
          frame #0 {
            n171 = Wait (ms)(milliseconds to wait=w662) -> ()  [unwired: 1 out]
            n172 = call <vilib>:"Serial Port Write.vi"("string to write"="_OXY\r" ("O2 partial press"), "port number"=w660) -> ()  [unwired: 1 out]
          }
          frame #1 {
            # "O2 partial pressure"
            n173 = call <vilib>:"Bytes At Serial Port.vi"() -> ("byte count"=w671:u32)  [unwired: 1 in, 1 out]
            n174 = Wait (ms)(milliseconds to wait=w670) -> ()  [unwired: 1 out]
            n175 = call <vilib>:"Serial Port Read.vi"("requested byte count"=w671, "port number"=w663) -> ("string read"=w669:string)  [unwired: 1 out]
            n176 = Fract/Exp String To Number(string=w669) -> (number=w667:dbl)  [unwired: 3 in, 1 out]
            "atm" <- w667
            n177 = Multiply(x=w667, y=100.0) -> (x*y=w664:dbl)
            "%" <- w664
            n178 = Multiply(x=w664, y=7.6) -> (x*y=w666:dbl)
            "Torr" <- w666
          }
        }
        n179 = Wait (ms)(milliseconds to wait=w647) -> ()  [unwired: 1 out]
        n180 = Greater?(x=w650, y=1e-07) -> (0:w653:bool)
        n181 = case shown="False" w653 {
          tunnel: [w658 w659] -> w652
          tunnel: w650 -> [_ w659]
          tunnel: w651 -> [w658 _]
          frame False {
          }
          frame True {
          }
        }
        n182 = Number To Engineering String(4:w652) -> (0:w648:string)  [unwired: 3 in]
        n183 = Bundle(w648) -> (w655:cluster{string})  [unwired: 1 in]
        n184 = Fract/Exp String To Number(string=w655) -> (number=→"Waveform Chart":cluster{dbl})  [unwired: 3 in, 1 out]
      }
    }
    n185 = Wait (ms)(milliseconds to wait=w261) -> ()  [unwired: 1 out]
    n186 = case "SRS QCM" shown="True" w282 {
      selector: w282 -> [w625 w631]
      tunnel: w285 -> [w629 w637]
      tunnel: w284 -> [w628 w639]
      tunnel: [w630 w644] -> w283
      tunnel: [w630 w643] -> w279
      tunnel: [w627 w642] -> w276
      tunnel: [0.0 w632] -> w241
      tunnel: [w625 w631] -> w249
      frame False {
        w630 = ""
        n187 = Bundle(w625, "VISA out"=w629, "error out"=w628) -> (w627:T7)  [unwired: 1 in]
      }
      frame True {
        # "SRS QCM"
        n188 = call "Elapsed Time2"() -> ("Elapsed Time (s)"=w638:dbl)  [unwired: 12 in, 7 out]
        n189 = call "SrsQcm200FandR_MODIFIED.vi"("VISA in"=w637, "Reference time in"=w638, "error in (no error)"=w639) -> ("VISA out"=w635:refnum<visa-resource-name>, "Frequency out"=w632:dbl, "Resistance out"=w634:dbl, "error out"=w636:errorcluster)  [unwired: 6 in, 3 out]
        "Ohm" <- w634
        n190 = Number To Engineering String(4:w634) -> (0:w643:string)  [unwired: 3 in]
        n191 = Divide(x=w632, y=1000000.0) -> (x/y=w633:dbl)
        "MHz" <- w633
        n192 = Number To Engineering String(4:w632) -> (0:w644:string)  [unwired: 3 in]
        n193 = Bundle(w633, "Resistance out"=w634) -> (→"Waveform Chart 7":cluster{dbl, "Resistance out":dbl})  [unwired: 1 in]
        n194 = Bundle(w631, "VISA out"=w635, "error out"=w636) -> (w642:T7)  [unwired: 1 in]
      }
    }
    n195 = case "Keithley 2420" shown="True" w258 {
      selector: w258 -> [w613 w621]
      tunnel: w287 -> [w612 w616]
      tunnel: w286 -> [w611 w615]
      tunnel: [w610 w619] -> w277
      tunnel: ["" w618] -> w278
      frame False {
        n196 = Bundle(w613, "VISA resource name out"=w612, "error out"=w611) -> (w610:T4)  [unwired: 1 in]
      }
      frame True {
        # "Keithley 2420"
        n197 = call-poly "Read.vi"("VISA resource name"=w616, "error in (no error)"=w615) -> ("VISA resource name out"=w622:refnum<visa-resource-name>, "Resistance"=w617:sgl, "error out"=w620:errorcluster)  [unwired: 7 in, 4 out]
        n198 = Bundle("Resistance"=w617) -> (→"Keithley 2420 (Ohm)":cluster{"Resistance":sgl})  [unwired: 1 in]
        n199 = Number To Engineering String(4:w617) -> (0:w618:string)  [unwired: 3 in]
        n200 = Wait (ms)(milliseconds to wait=u32 20) -> ()  [unwired: 1 out]
        n201 = Bundle(w621, "VISA resource name out"=w622, "error out"=w620) -> (w619:T4)  [unwired: 1 in]
      }
    }
    n202 = case "Keithley 6430" shown="True" w251 {
      selector: w251 -> [w516 w526]
      tunnel: w254 -> [w515 w523]
      tunnel: w253 -> [w514 w522]
      tunnel: ["" w525] -> w213
      tunnel: [w513 w524] -> w252
      frame False {
        n203 = Bundle(w516, "VISA resource name out"=w515, "error out"=w514) -> (w513:T4)  [unwired: 1 in]
      }
      frame True {
        # "Keithley 6430"
        n204 = call-poly "Read.vi"("error in (no error)"=w522, "VISA resource name"=w523) -> ("error out"=w521:errorcluster, "Measurement"=w519:dbl, "VISA resource name out"=w520:refnum<visa-resource-name>)  [unwired: 1 in, 6 out]
        n205 = Number To Engineering String(4:w519) -> (0:w525:string)  [unwired: 3 in]
        n206 = Bundle("Measurement"=w519) -> (→"Keithley 6430 (Ohm)":cluster{"Measurement":dbl})  [unwired: 1 in]
        n207 = Wait (ms)(milliseconds to wait=u32 20) -> ()  [unwired: 1 out]
        n208 = Bundle(w526, "VISA resource name out"=w520, "error out"=w521) -> (w524:T4)  [unwired: 1 in]
      }
    }
    n209 = Unbundle(w267) -> (w266:bool, "VISA resource name out"=w265:refnum<visa-resource-name>, "error out"=w264:errorcluster)
    n210 = Greater?(x=w204, y=1.0) -> (0:w214:bool)
    n211 = case "RapidOX O2 Sensor" shown="True" w266 {
      tunnel: w265 -> [_ w537]
      tunnel: w264 -> [w530 w536]
      tunnel: ["" w535] -> w263
      tunnel: [w530 w532] -> w262
      frame False {
      }
      frame True {
        # "RapidOX 2100"
        n212 = VISA Write(VISA resource name=w537, write buffer="D", error in (no error)=w536) -> (VISA resource name out=w540:refnum<visa-resource-name>, error out=w539:errorcluster)  [unwired: 1 out]
        n213 = flat-sequence {
          tunnel: [w549] -> w546
          tunnel: [w547] -> w545
          tunnel: w540 -> [w549]
          tunnel: w539 -> [w547]
          tunnel: w546 -> [w554]
          tunnel: w545 -> [w553]
          tunnel: [w552] -> w544
          tunnel: [w551] -> w543
          tunnel: [w550] -> w542
          tunnel: w544 -> [w563]
          tunnel: w543 -> [w562]
          tunnel: w542 -> [w561]
          tunnel: [w560] -> w532
          tunnel: [w555] -> w534
          frame #0 {
            n214 = Wait (ms)(milliseconds to wait=u32 100) -> ()  [unwired: 1 out]
          }
          frame #1 {
            n215 = property class="Instr"(reference=w554, error in=w553) -> (reference out=w552:refnum<visa-resource-name>, error out=w550:errorcluster, "Bytes at Port"=w551:u32)
          }
          frame #2 {
            n216 = VISA Read(VISA resource name=w563, byte count=w562, error in (no error)=w561) -> (read buffer=w558:string, error out=w560:errorcluster)  [unwired: 2 out]
            n217 = Match Pattern(string=w558, regular expression="d") -> (after substring=w556:string)  [unwired: 1 in, 3 out]
            n218 = Match Pattern(string=w556, regular expression=",") -> (before substring=w555:string)  [unwired: 1 in, 3 out]
          }
        }
        n219 = flat-sequence {
          frame #0 {
          }
        }
        n220 = Fract/Exp String To Number(string=w534) -> (number=w533:dbl)  [unwired: 3 in, 1 out]
        "O2 Concentration (PPM)" <- w533
        n221 = Bundle(w533) -> (→"Waveform Chart 6":cluster{dbl})  [unwired: 1 in]
        n222 = Number To Engineering String(4:w533) -> (0:w535:string)  [unwired: 3 in]
      }
    }
    n223 = And(x=w214, y=w215) -> (x .and. y?=w226:bool)
    n224 = case shown="True" w226 {
      selector: w226 -> [w294 w325]
      tunnel: w225 -> [w296 w304]
      tunnel: w224 -> [w295 w305]
      tunnel: [w296 w308] -> w222
      tunnel: [w295 w307] -> w221
      tunnel: [w294 w325] -> w223
      tunnel: [w293 w306] -> w220
      tunnel: [w293 w299] -> w216
      tunnel: [w293 w303] -> w217
      frame False {
        w293 = ""
      }
      frame True {
        n225 = property class="Instr"(reference=w304, error in=w305) -> (reference out=w322:refnum<visa-resource-name>, error out=w324:errorcluster, "Bytes at Port"=w323:u32)
        n226 = VISA Read(VISA resource name=w322, byte count=w323, error in (no error)=w324) -> (VISA resource name out=w308:refnum<visa-resource-name>, read buffer=w297:string, error out=w307:errorcluster)  [unwired: 1 out]
        n227 = flat-sequence {
          tunnel: [w327] -> w298
          tunnel: w297 -> [w327]
          frame #0 {
            n228 = Wait (ms)(milliseconds to wait=u32 1500) -> ()  [unwired: 1 out]
          }
        }
        n229 = Search/Split String(string=w298, search string/char (-)=":") -> (match + rest of string=w319:string)  [unwired: 1 in, 2 out]
        n230 = Search/Split String(string=w319, offset (0)=1) -> (match + rest of string=w317:string)  [unwired: 1 in, 2 out]
        n231 = Search/Split String(string=w317, search string/char (-)="h") -> (substring before match=w306:string, match + rest of string=w315:string)  [unwired: 1 in, 1 out]
        "gas\nsensor" <- w306
        n232 = Search/Split String(string=w315, offset (0)=2) -> (match + rest of string=w313:string)  [unwired: 1 in, 2 out]
        n233 = Search/Split String(string=w313, search string/char (-)="t") -> (substring before match=w303:string, match + rest of string=w311:string)  [unwired: 1 in, 1 out]
        n234 = Search/Split String(string=w311, offset (0)=2) -> (match + rest of string=w301:string)  [unwired: 1 in, 2 out]
        n235 = Fract/Exp String To Number(string=w303) -> (number=w309:dbl)  [unwired: 3 in, 1 out]
        n236 = Bundle(w309) -> (→"Arduino humidity (%)":cluster{dbl})  [unwired: 1 in]
        n237 = Search/Split String(string=w301, search string/char (-)=".", offset (0)=0) -> (substring before match=w299:string)  [unwired: 2 out]
        "temp\n(C)" <- w299
      }
    }
    n238 = Select(t=w241, s=w243, f=w242) -> (s? t:f=w240:dbl)
    n239 = case shown="True" w249 {
      tunnel: w241 -> [_ w510]
      tunnel: ["" w508] -> w255
      tunnel: w240 -> [_ w507]
      frame False {
      }
      frame True {
        n240 = Subtract(x=w507, y=w510) -> (x-y=w511:dbl)
        n241 = Divide(x=w511, y=56.65) -> (x/y=w506:dbl)
        n242 = Bundle(w506) -> (→"QCM mass deposited (ug)":cluster{dbl})  [unwired: 1 in]
        n243 = Number To Engineering String(4:w506) -> (0:w508:string)  [unwired: 3 in]
      }
    }
    n244 = Get Date/Time In Seconds() -> (seconds since 1Jan1904=w292:timestamp)
    n245 = Format Date/Time String(time format string (%c)="%Y-%m-%d %H:%M:%S%2u", seconds (now)=w292) -> (date/time string=w288:string)  [unwired: 1 in]
    n246 = Build Array(w288, w291, w213, w272, w278, w255, w283, w279, w280, w263, w239, w205, w238, w237, w220, w217, w216) -> (w219:string[])
  }
  n247 = Unbundle(w80) -> (w79:bool, "VISA resource name out"=w78:refnum<visa-resource-name>, "error out"=w77:errorcluster)
  n248 = Unbundle(w85) -> (w84:bool, "VISA out"=w83:refnum<visa-resource-name>, "error out"=w82:errorcluster)
  n249 = Unbundle(w89) -> (w88:bool, "VISA resource name out"=w87:refnum<visa-resource-name>, "error out"=w86:errorcluster)
  n250 = case shown="True" w26 {
    tunnel: w25 -> [_ w673]
    tunnel: w24 -> [_ w672]
    frame False {
    }
    frame True {
      n251 = VISA Close(VISA resource name=w673, error in (no error)=w672) -> ()  [unwired: 1 out]
    }
  }
  n252 = Unbundle(w51) -> (w56:bool, "VISA resource name out"=w55:refnum<visa-resource-name>, "error out"=w54:errorcluster)
  n253 = case shown="True" w43 {
    tunnel: [w674 w694] -> w41
    tunnel: w44 -> [_ w693]
    tunnel: w45 -> [_ w692]
    tunnel: w47 -> [_ w688]
    tunnel: w46 -> [_ w687]
    tunnel: [w674 w686] -> w42
    tunnel: [w675 w683] -> w40
    tunnel: w38 -> [w675 w682]
    tunnel: w30 -> [_ w679]
    tunnel: [w674 w678] -> w33
    tunnel: w32 -> [_ w677]
    tunnel: w31 -> [_ w676]
    frame False {
      w674 = errorcluster {"status"=FALSE, "code"=0, "source"=""} ("error out")
    }
    frame True {
      n254 = call <vilib>:"DAQmx Stop Task.vi"("task/channels in"=w677, "error in"=w676) -> ("task out"=w680:refnum<k21>, "error out"=w681:errorcluster)  [unwired: 12 in]
      n255 = call <vilib>:"DAQmx Stop Task.vi"("task/channels in"=w688, "error in"=w687) -> ("task out"=w690:refnum<k21>, "error out"=w689:errorcluster)  [unwired: 12 in]
      n256 = call <vilib>:"DAQmx Stop Task.vi"("task/channels in"=w693, "error in"=w692) -> ("task out"=w691:refnum<k21>, "error out"=w695:errorcluster)  [unwired: 12 in]
      n257 = VISA Clear(VISA resource name=w679, error in (no error)=w682) -> (VISA resource name out=w685:refnum<visa-resource-name>, error out=w684:errorcluster)
      n258 = call <vilib>:"DAQmx Clear Task.vi"("task in"=w680, "error in"=w681) -> ("error out"=w678:errorcluster)  [unwired: 13 in]
      n259 = call <vilib>:"DAQmx Clear Task.vi"("task in"=w690, "error in"=w689) -> ("error out"=w686:errorcluster)  [unwired: 13 in]
      n260 = call <vilib>:"DAQmx Clear Task.vi"("task in"=w691, "error in"=w695) -> ("error out"=w694:errorcluster)  [unwired: 13 in]
      n261 = VISA Close(VISA resource name=w685, error in (no error)=w684) -> (error out=w683:errorcluster)
    }
  }
  n262 = case shown="True" w88 {
    tunnel: w87 -> [_ w699]
    tunnel: w86 -> [w696 w698]
    tunnel: [w696 w697] -> w90
    frame False {
    }
    frame True {
      n263 = call "Enable Output.vi"("error in (no error)"=w698, "Enable Output (T: Enable)"=FALSE, "VISA resource name"=w699) -> ("error out"=w700:errorcluster, "VISA resource name out"=w702:refnum<visa-resource-name>)  [unwired: 7 in]
      n264 = call "Close.vi"("error in (no error)"=w700, "VISA resource name"=w702) -> ("error out"=w697:errorcluster)  [unwired: 9 in]
    }
  }
  n265 = case shown="True" w56 {
    tunnel: w55 -> [_ w705]
    tunnel: w54 -> [w703 w704]
    tunnel: [w703 w706] -> w50
    frame False {
    }
    frame True {
      w709 = FALSE  # Output (F:Off)
      n266 = call "Enable Output.vi"("error in (no error)"=w704, "Enable Output (F:Off)"=w709, "VISA resource name"=w705) -> ("error out"=w707:errorcluster, "VISA resource name out"=w708:refnum<visa-resource-name>)  [unwired: 7 out]
      n267 = call "Close.vi"("error in (no error)"=w707, "VISA resource name"=w708) -> ("error out"=w706:errorcluster)  [unwired: 9 out]
    }
  }
  n268 = case shown="False" w84 {
    tunnel: w82 -> [w710 w713]
    tunnel: [w710 w712] -> w91
    tunnel: w83 -> [_ w711]
    frame False {
    }
    frame True {
      n269 = call "srsQcm200Close.vi"("error in"=w713, "Visa in"=w711) -> ("error out"=w712:errorcluster)  [unwired: 3 in]
    }
  }
  n270 = case shown="True" w79 {
    tunnel: w78 -> [_ w717]
    tunnel: w77 -> [w714 w716]
    tunnel: [w714 w715] -> w76
    frame False {
    }
    frame True {
      n271 = VISA Close(VISA resource name=w717, error in (no error)=w716) -> (error out=w715:errorcluster)
    }
  }
  n272 = Merge Errors(w33, w42, w41, w40) -> (w39:errorcluster)
  n273 = Merge Errors(w50, w76, w90, w91, w61, w39) -> (w98:errorcluster)
  n274 = call <vilib>:"Simple Error Handler.vi"("error in (no error)"=w98) -> ()  [unwired: 4 in, 5 out]
  n275 = Build Array("date/time", "min elapsed", "Keithley 6430 resistance (Ohm)", "J-KEM temp (C)", "Keithley 2420 resistance (Ohm)" ("element"), "QCM adsorbed mass (ug)", "QCM freq (Hz)", "QCM resistance (Ohm)", "O2 partial pressure (Torr)" ("element"), "O2 concentration (PPM)" ("element"), "chamber pressure (Torr)" ("element"), "chamber RH (%)" ("element"), "gas flow (sccm)" ("element"), "vapor flow (sccm)" ("element"), "gas sensor" ("element"), "humidity (%)" ("element"), "temp (C)" ("element"), "Experiment Notes") -> (w68:string[])
  n276 = call-poly <vilib>:"Write To Spreadsheet File.vi"("1D data"=w68, "file path (dialog if empty)"=w60) -> ("new file path (Not A Path if cancelled)"=w69:path)  [unwired: 6 in]
  n277 = call-poly <vilib>:"Write To Spreadsheet File.vi"("append to file? (new file:F)"=TRUE, "2D data"=w97, "file path (dialog if empty)"=w69) -> ()  [unwired: 5 in, 1 out]
